vi "ScansteuerungZuPixelinfo_withBorder.vi"(6 "error in (no error)":errorcluster, 8 "ScanSteuerung":T1(array[cluster])=[{"Zeitpunkt [s]"=0.0, "Wirkung"=enum."Abs", "Kanal"=enum."SMoveTime", "Wert (/s)"=0.00096}, {"Zeitpunkt [s]"=0.0, "Wirkung"=enum."Abs", "Kanal"=enum."GalvoX", "Wert (/s)"=-0.0005171784141124036}, {"Zeitpunkt [s]"=0.0, "Wirkung"=enum."Abs", "Kanal"=enum."GalvoY", "Wert (/s)"=-0.0005424121424136167}, {"Zeitpunkt [s]"=0.0, "Wirkung"=enum."Abs", "Kanal"=enum."Galvo3", "Wert (/s)"=0.0}, {"Zeitpunkt [s]"=0.0, "Wirkung"=enum."Abs", "Kanal"=enum."Image1X", "Wert (/s)"=0.0}, {"Zeitpunkt [s]"=0.0, "Wirkung"=enum."Abs", "Kanal"=enum."Image1Y", "Wert (/s)"=0.0}, {"Zeitpunkt [s]"=0.0, "Wirkung"=enum."Abs", "Kanal"=enum."Digital", "Wert (/s)"=2.0}, {"Zeitpunkt [s]"=0.0, "Wirkung"=enum."LoopStart", "Kanal"=enum."Loop", "Wert (/s)"=250.0}, {"Zeitpunkt [s]"=0.0, "Wirkung"=enum."Inc", "Kanal"=enum."GalvoX", "Wert (/s)"=0.0833334166669957}, {"Zeitpunkt [s]"=0.0, "Wirkung"=enum."Inc", "Kanal"=enum."GalvoY", "Wert (/s)"=0.0}, {"Zeitpunkt [s]"=2.4e-05, "Wirkung"=enum."Inc", "Kanal"=enum."Image1X", "Wert (/s)"=41666.666666666664}, {"Zeitpunkt [s]"=0.011976, "Wirkung"=enum."Abs", "Kanal"=enum."Digital", "Wert (/s)"=3.0}, {"Zeitpunkt [s]"=0.011976, "Wirkung"=enum."Inc", "Kanal"=enum."GalvoX", "Wert (/s)"=0.0}, {"Zeitpunkt [s]"=0.011976, "Wirkung"=enum."Inc", "Kanal"=enum."GalvoY", "Wert (/s)"=0.04166670833349785}, {"Zeitpunkt [s]"=0.011976, "Wirkung"=enum."Inc", "Kanal"=enum."Image1X", "Wert (/s)"=0.0}, {"Zeitpunkt [s]"=0.012048, "Wirkung"=enum."Abs", "Kanal"=enum."Digital", "Wert (/s)"=2.0}, {"Zeitpunkt [s]"=0.012048, "Wirkung"=enum."Rel", "Kanal"=enum."Image1Y", "Wert (/s)"=1.0}, {"Zeitpunkt [s]"=0.012048, "Wirkung"=enum."Inc", "Kanal"=enum."GalvoX", "Wert (/s)"=-0.0833334166669957}, {"Zeitpunkt [s]"=0.012048, "Wirkung"=enum."Inc", "Kanal"=enum."GalvoY", "Wert (/s)"=-0.0}, {"Zeitpunkt [s]"=0.012096, "Wirkung"=enum."Inc", "Kanal"=enum."Image1X", "Wert (/s)"=-41666.666666666664}, {"Zeitpunkt [s]"=0.024048, "Wirkung"=enum."Abs", "Kanal"=enum."Digital", "Wert (/s)"=3.0}, {"Zeitpunkt [s]"=0.024048, "Wirkung"=enum."Inc", "Kanal"=enum."GalvoX", "Wert (/s)"=0.0}, {"Zeitpunkt [s]"=0.024048, "Wirkung"=enum."Inc", "Kanal"=enum."GalvoY", "Wert (/s)"=0.04166670833349785}, {"Zeitpunkt [s]"=0.024048, "Wirkung"=enum."Inc", "Kanal"=enum."Galvo3", "Wert (/s)"=0.0}, {"Zeitpunkt [s]"=0.024048, "Wirkung"=enum."Inc", "Kanal"=enum."Image1X", "Wert (/s)"=0.0}, {"Zeitpunkt [s]"=0.024096, "Wirkung"=enum."Abs", "Kanal"=enum."Digital", "Wert (/s)"=2.0}, {"Zeitpunkt [s]"=0.024096, "Wirkung"=enum."Rel", "Kanal"=enum."Image1Y", "Wert (/s)"=1.0}, {"Zeitpunkt [s]"=0.024096, "Wirkung"=enum."LoopEnd", "Kanal"=enum."Loop", "Wert (/s)"=0.0}, {"Zeitpunkt [s]"=6.024, "Wirkung"=enum."Inc", "Kanal"=enum."GalvoX", "Wert (/s)"=0.0}, {"Zeitpunkt [s]"=6.024, "Wirkung"=enum."Inc", "Kanal"=enum."GalvoY", "Wert (/s)"=0.0}, {"Zeitpunkt [s]"=6.024, "Wirkung"=enum."Inc", "Kanal"=enum."Galvo3", "Wert (/s)"=0.0}, {"Zeitpunkt [s]"=6.024, "Wirkung"=enum."Abs", "Kanal"=enum."Digital", "Wert (/s)"=0.0}]) -> (0 "error out":errorcluster, 1 "Pixelindex":u32[](array[numeric]), 2 "Pixelzeit in s":dbl=12.0 min=0.4 max=10000.0 step=0.05, 3 "TotalPixels (incl. turn)":i32=8, 4 "ypixels":u32=10, 5 "xPixels":u32=1000)   [LabVIEW 2011]
panel:
  out "data/line":u32
  out "Err":bool
  # "add alignment to have multipe of 16 in x, not tested so far!"
  # "this example dataset is bad!!"
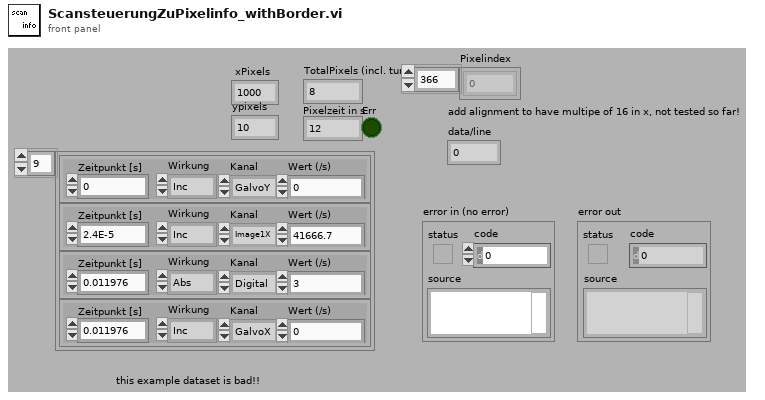
[diagram p1: front panel]
types:
  T1 = cluster{"Zeitpunkt [s]":dbl, "Wirkung":enum16{"Abs", "Rel", "Inc", "IncInc", "LoopStart", "LoopEnd"}, "Kanal":enum16{"Com", "AnalogConfig", "AnalogValue", "GalvoX", "GalvoY", "Galvo3", "Galvo4", "Digital", "Free", "Loop", "SMoveTime", "Image1X", "Image1Y", "Image2X", "Image2Y"}, "Wert (/s)":dbl}[]
  T2 = enum16{"Com", "AnalogConfig", "AnalogValue", "GalvoX", "GalvoY", "Galvo3", "Galvo4", "Digital", "Free", "Loop", "SMoveTime", "Image1X", "Image1Y", "Image2X", "Image2Y"}
  T3 = enum16{"Com", "AnalogConfig", "AnalogValue", "GalvoX", "GalvoY", "Galvo3", "Galvo4", "Digital", "Free", "Loop", "SMoveTime", "Image1X", "Image1Y", "Image2X", "Image2Y"}[]
  T4 = typedef "ScanControl.ctl" = cluster{"Time [s]":dbl, "action":T5, "channel":T6, "value (/s)":dbl}[]
  T5 = typedef "ScanControl_Action.ctl" = enum16{"Abs", "Rel", "Inc", "IncInc", "LoopStart", "LoopEnd", "WaitTriggerRising"}
  T6 = typedef "ScanControl_Channel.ctl" = enum16{"Com", "AnalogConfig", "AnalogValue", "GalvoX", "GalvoY", "Galvo3", "Galvo4", "Digital", "Free", "Loop", "SMoveTime", "Image1X", "Image1Y", "Image2X", "Image2Y"}
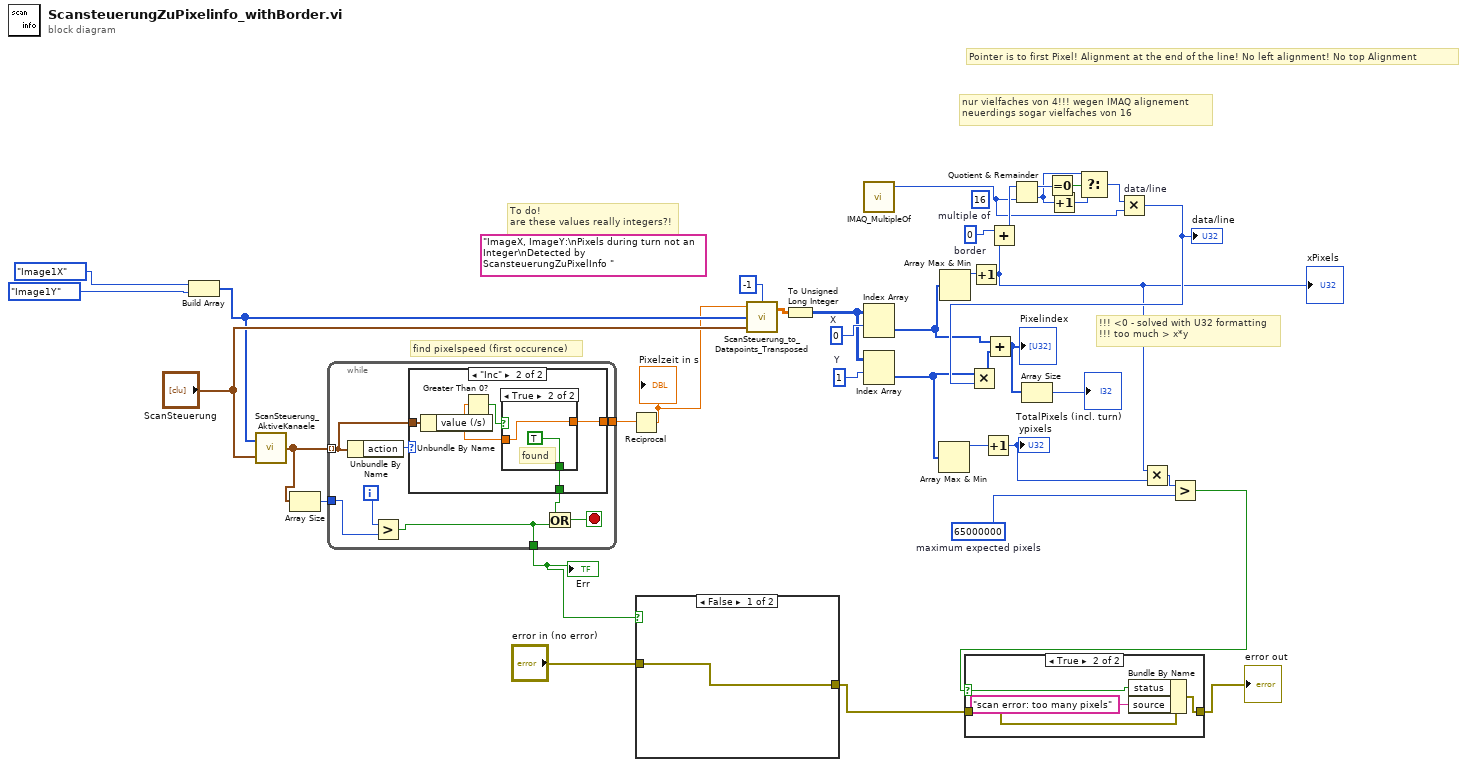
[diagram p0: block diagram]
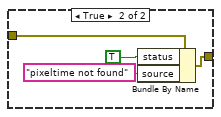
[diagram p3: hidden frame]
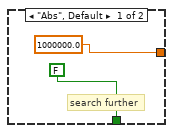
[diagram p4: hidden frame]
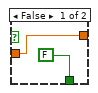
[diagram p5: hidden frame]
diagram:
  w7 = u32 65000000  # maximum expected pixels
  w20 = u32 0  # border
  (unwired) u32 16  # multiple of
  (unwired) "ImageX, ImageY:\nPixels during turn not an Integer\nDetected by ScansteuerungZuPixelInfo " ("source")
  w18 = 1  # Y
  w19 = 0  # X
  # "Pointer is to first Pixel! Alignment at the end of the line! No left alignment! No top Alignment"
  # "nur vielfaches von 4!!! wegen IMAQ alignement\nneuerdings sogar vielfaches von 16"
  # "To do!\nare these values really integers?!"
  # "!!! <0 - solved with U32 formatting\n!!! too much > x*y"
  # "find pixelspeed (first occurence)"
  n1 = Build Array(T2."Image1X" ("Kanal"), T2."Image1Y" ("Kanal")) -> (w28:T3)
  n2 = call "ScanSteuerung_AktiveKanaele.vi"("ScanSteuerung"="ScanSteuerung", "Aktiv"=w28) -> ("ScanSteuerungOut"=w32:T4)
  n3 = Array Size(array=w32) -> (size(s)=w31:i32)
  n4 = while {
    tunnel: w32 -> [w45] mode=indexing
    tunnel: [w44] -> w35
    tunnel: w31 -> [w41]
    tunnel: [w39] -> w26
    i -> [w42]
    stop <- w40 stop-if-true
    n5 = Unbundle By Name(w45) -> ("action"=w46:T5)
    n6 = Greater?(x=w42, y=w41) -> (0:w39:bool)
    n7 = case shown="\"Inc\"" w46 {
      tunnel: w45 -> [_ w53]
      tunnel: [1000000.0 w50] -> w44
      tunnel: [FALSE w49] -> w43
      frame "Abs", Default {
        # "search further"
      }
      frame "Inc" {
        n8 = Unbundle By Name(w53) -> ("value (/s)"=w51:dbl)
        n9 = Greater Than 0?(x=w51) -> (x > 0?=w52:bool)
        n10 = case shown="True" w52 {
          tunnel: w51 -> [w54 w57]
          tunnel: [w54 w57] -> w50
          tunnel: [FALSE TRUE] -> w49
          frame False {
          }
          frame True {
            # "found"
          }
        }
      }
    }
    n11 = Or(x=w43, y=w39) -> (x .or. y?=w40:bool)
  }
  "Err" <- w26
  n12 = Reciprocal(x=w35) -> (1/x=w27:dbl)
  "Pixelzeit in s" <- w27
  n13 = case shown="False" w26 {
    tunnel: "error in (no error)" -> [w58 w62]
    tunnel: [w58 w61] -> w6
    frame False {
    }
    frame True {
      n14 = Bundle By Name(cluster=w62, "status"=TRUE, "source"="pixeltime not found") -> (w61:errorcluster)
    }
  }
  n15 = call "ScanSteuerung_to_Datapoints_Transposed.vi"("Datapoints (-1=estimate)"=-1, "ScanSteuerung"="ScanSteuerung", "Aktiv"=w28, "Neues Zeitraster"=w27) -> ("Waveform Graph"=w29:dbl[][])  [unwired: 1 out]
  n16 = To Unsigned Long Integer(number=w29) -> (unsigned 32bit integer=w11:u32[][])
  n17 = call "IMAQ_MultipleOf.vi"() -> ("LineWidthMultipleOf"=w8:i32)  [unwired: 3 out]
  n18 = Index Array(array=w11, index (row)=w19) -> (element=w10:u32[])  [unwired: 1 in]
  n19 = Index Array(array=w11, index (row)=w18) -> (element=w9:u32[])  [unwired: 1 in]
  n20 = Array Max & Min(array=w9) -> (max value=w34:u32)  [unwired: 3 out]
  n21 = Array Max & Min(array=w10) -> (max value=w33:u32)  [unwired: 3 out]
  n22 = Increment(x=w33) -> (x+1=w4:u32)
  "xPixels" <- w4
  n23 = Increment(x=w34) -> (x+1=w3:u32)
  "ypixels" <- w3
  n24 = Add(x=w20, y=w4) -> (x+y=w17:u32)
  n25 = Quotient & Remainder(x=w17, y=w8) -> (x-y*floor(x/y)=w15:u32, floor(x/y)=w14:u32)
  n26 = Equal To 0?(x=w15) -> (x = 0?=w16:bool)
  n27 = Increment(x=w14) -> (x+1=w13:u32)
  n28 = Select(t=w14, s=w16, f=w13) -> (s? t:f=w12:u32)
  n29 = Multiply "data/line"(x=w12, y=w8) -> (x*y=w21:u32)
  "data/line" <- w21
  n30 = Multiply(x=w9, y=w21) -> (x*y=w38:u32[])
  n31 = Add(x=w10, y=w38) -> (x+y=w37:u32[])
  "Pixelindex" <- w37
  n32 = Array Size(array=w37) -> (size(s)=→"TotalPixels (incl. turn)":i32)
  n33 = Multiply(x=w4, y=w3) -> (x*y=w2:u32)
  n34 = Greater?(x=w2, y=w7) -> (0:w1:bool)
  n35 = case shown="True" w1 {
    selector: w1 -> [_ w66]
    tunnel: w6 -> [w63 w67]
    tunnel: [w63 w65] -> w5
    frame False {
    }
    frame True {
      n36 = Bundle By Name(cluster=w67, "status"=w66, "source"="scan error: too many pixels") -> (w65:errorcluster)
    }
  }
  "error out" <- w5
